vi "config.vi"(8 "error in (no error)":errorcluster, 10 "Configuration":T2={"Config Dir"=path "/home/ttsai/Documents/stash/ts_tcs_ofc/configData", "Inst Name"=enum."lsst", "Config File Name"="pinv.esti", "Mapping File Name"="sensorNameToFieldIdx.txt", "Wavelength Table"="effWaveLength.txt", "Intrinc Zk File Name"="intrinsic_zn", "y2 Corection File Name"="y2.txt"}, 11 "OptStateEsti in":refnum<class "OptStateEsti.lvclass">) -> (0 "error out":errorcluster, 3 "OptStateEsti out":refnum<class "OptStateEsti.lvclass">)   [LabVIEW 2016, in "OptStateEsti.lvclass"]
doc: "Do the configuration of optical state estimator (OSE)."
uses:
  OptStateEsti.lvclass
  StrictDef/InstName.ctl
  OptStateEsti.lvclass/OptStateEsti.ctl
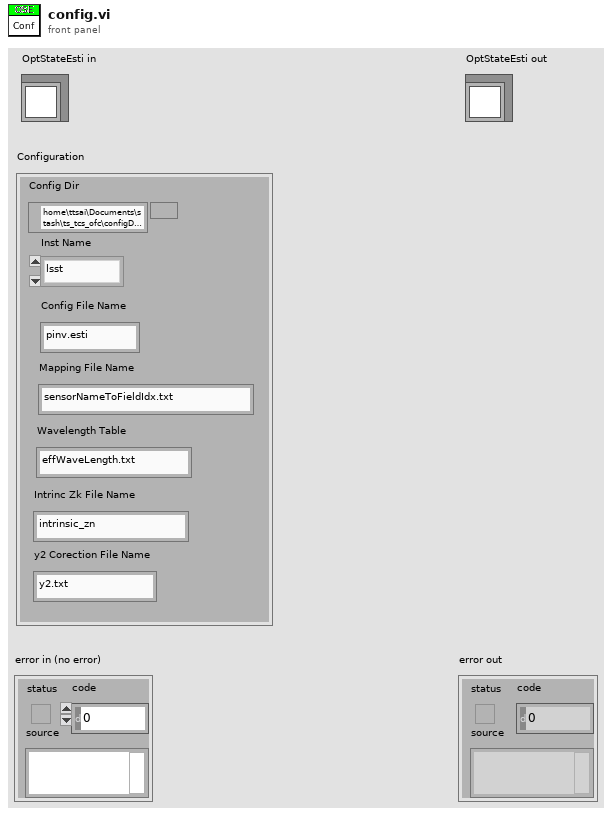
[diagram p1: front panel]
types:
  T1 = typedef "InstName.ctl" = enum16{"lsst", "comcam"}
  T2 = cluster{"Config Dir":path, "Inst Name":T1, "Config File Name":string, "Mapping File Name":string, "Wavelength Table":string, "Intrinc Zk File Name":string, "y2 Corection File Name":string}
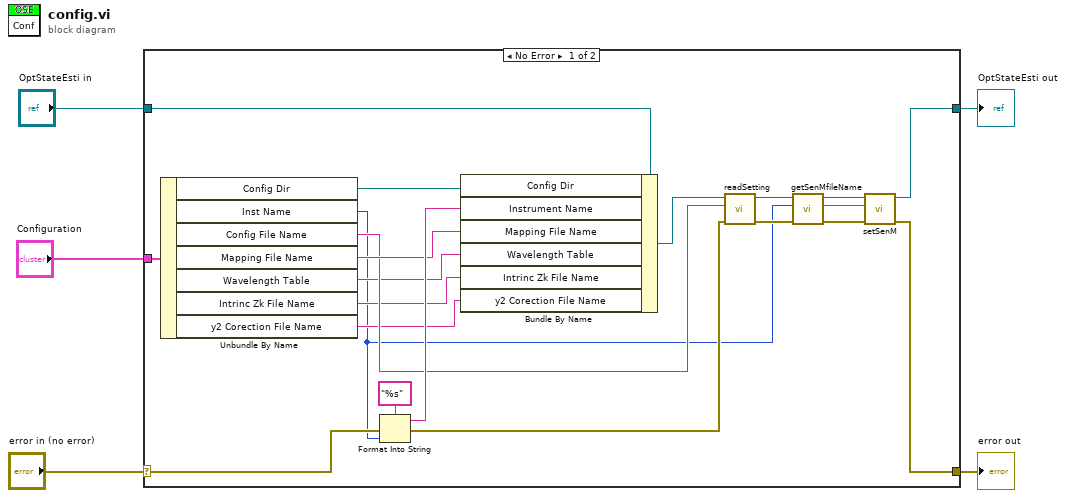
[diagram p0: block diagram]
diagram:
  n1 = case shown="No Error" "error in (no error)" {
    selector: "error in (no error)" -> [w24 w28]
    tunnel: [w13 w28] -> w4
    tunnel: [w14 w27] -> w2
    tunnel: "OptStateEsti in" -> [w23 w27]
    tunnel: "Configuration" -> [w26 _]
    frame No Error {
      n2 = Unbundle By Name(w26) -> ("Config Dir"=w22:path, "Inst Name"=w6:T1, "Config File Name"=w19:string, "Mapping File Name"=w20:string, "Wavelength Table"=w18:string, "Intrinc Zk File Name"=w17:string, "y2 Corection File Name"=w16:string)
      n3 = Format Into String(format string="%s", error in=w24, w6) -> (resulting string=w21:string, error out=w12:errorcluster)  [unwired: 1 in]
      n4 = Bundle By Name(cluster=w23, "Config Dir"=w22, "Instrument Name"=w21, "Mapping File Name"=w20, "Wavelength Table"=w18, "Intrinc Zk File Name"=w17, "y2 Corection File Name"=w16) -> (w15:refnum<class "OptStateEsti.lvclass">)
      n5 = call "readSetting.vi"("error in (no error)"=w12, "Config File Name"=w19, "OptStateEsti in"=w15) -> ("error out"=w10:errorcluster, "OptStateEsti out"=w11:refnum<class "OptStateEsti.lvclass">)  [unwired: 7 in]
      n6 = call "getSenMfileName.vi"("error in (no error)"=w10, "Inst Name"=w6, "OptStateEsti in"=w11) -> ("error out"=w8:errorcluster, "Sen M File Name"=w9:string, "OptStateEsti out"=w7:refnum<class "OptStateEsti.lvclass">)  [unwired: 6 in]
      n7 = call "setSenM.vi"("error in (no error)"=w8, "Sen M File Name"=w9, "OptStateEsti in"=w7) -> ("error out"=w13:errorcluster, "OptStateEsti out"=w14:refnum<class "OptStateEsti.lvclass">)  [unwired: 7 in]
    }
    frame Error {
    }
  }
  "error out" <- w4
  "OptStateEsti out" <- w2
